vi "Configure ADC.vi"(8 "error in (no error)":errorcluster, 9 "Gain Values":T1, 10 "Sample Rate":T2=128 items=["128Hz"=0, "250Hz"=32, "490Hz"=64, "920Hz"=96, "1600Hz"=128, "2400Hz"=160, "3300Hz"=192], 11 "ExplorerHatPro in":refnum<class "LINX-ExplorerHatPro.lvclass">) -> (0 "error out":errorcluster, 3 "ExplorerHatPro out":refnum<class "LINX-ExplorerHatPro.lvclass">)   [LabVIEW 2020, in "LINX-ExplorerHatPro.lvclass"]
uses:
  LINX-ExplorerHatPro.lvclass
  LINX-ExplorerHatPro.lvclass/LINX-ExplorerHatPro.ctl
  Read ADS1015.vi
  Write ADS1015.vi
  LINX-ADS1015/LINX-ADS1X15.lvclass
  LINX-ADS1015/ADS1015 Sample Rate.ctl
  LINX-ADS1015/Programmable Gain Selection.ctl
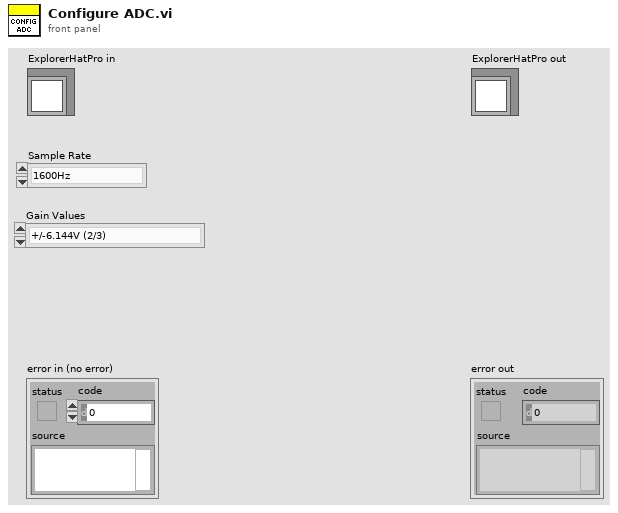
[diagram p1: front panel]
types:
  T1 = typedef "LINX-ADS1X15.lvclass/Programmable Gain Selection.ctl" = enum16{"+/-6.144V (2/3)", "+/-4.096V (1)", "+/-2.048V (2)", "+/-1.024V (4)", "+/-0.512V (8)", "+/-0.256V (16)"}
  T2 = typedef "LINX-ADS1X15.lvclass/ADS1015 Sample Rate.ctl" = u16
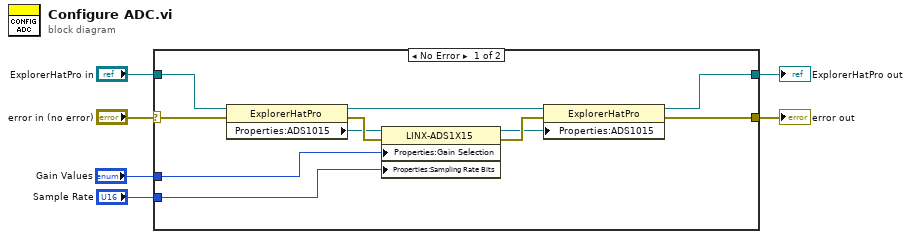
[diagram p0: block diagram]
diagram:
  n1 = case shown="No Error" "error in (no error)" {
    selector: "error in (no error)" -> [w15 w18]
    tunnel: [w11 w18] -> w5
    tunnel: [w13 w17] -> w3
    tunnel: "ExplorerHatPro in" -> [w16 w17]
    tunnel: "Gain Values" -> [w8 _]
    tunnel: "Sample Rate" -> [w7 _]
    frame No Error {
      n2 = property class="ExplorerHatPro"(reference=w16, error in=w15) -> (reference out=w13:refnum<class "LINX-ExplorerHatPro.lvclass">, error out=w14:errorcluster, "Properties:ADS1015"=w10:refnum<class "LINX-ADS1X15.lvclass">)
      n3 = property class="LINX-ADS1X15"(reference=w10, error in=w14, "Properties:Gain Selection"=w8, "Properties:Sampling Rate Bits"=w7) -> (reference out=w9:refnum<class "LINX-ADS1X15.lvclass">, error out=w12:errorcluster)
      n4 = property class="ExplorerHatPro"(reference=w13, error in=w12, "Properties:ADS1015"=w9) -> (error out=w11:errorcluster)  [unwired: 1 out]
    }
    frame Error {
    }
  }
  "error out" <- w5
  "ExplorerHatPro out" <- w3
